vi "QuickDrop Read QDKS INI Info.vi"(8 "error in":errorcluster, 11 "Mappings from INI":string) -> (0 "error out":errorcluster, 1 "All Plugin Paths":path[](array[path]), 2 "INI Names":string[](array[string]), 3 "INI Configured Shortcuts":string[](array[string]))   [LabVIEW 2020]
uses:
  <vilib>/Utility/lvfile.llb/NI_FileType.lvlib
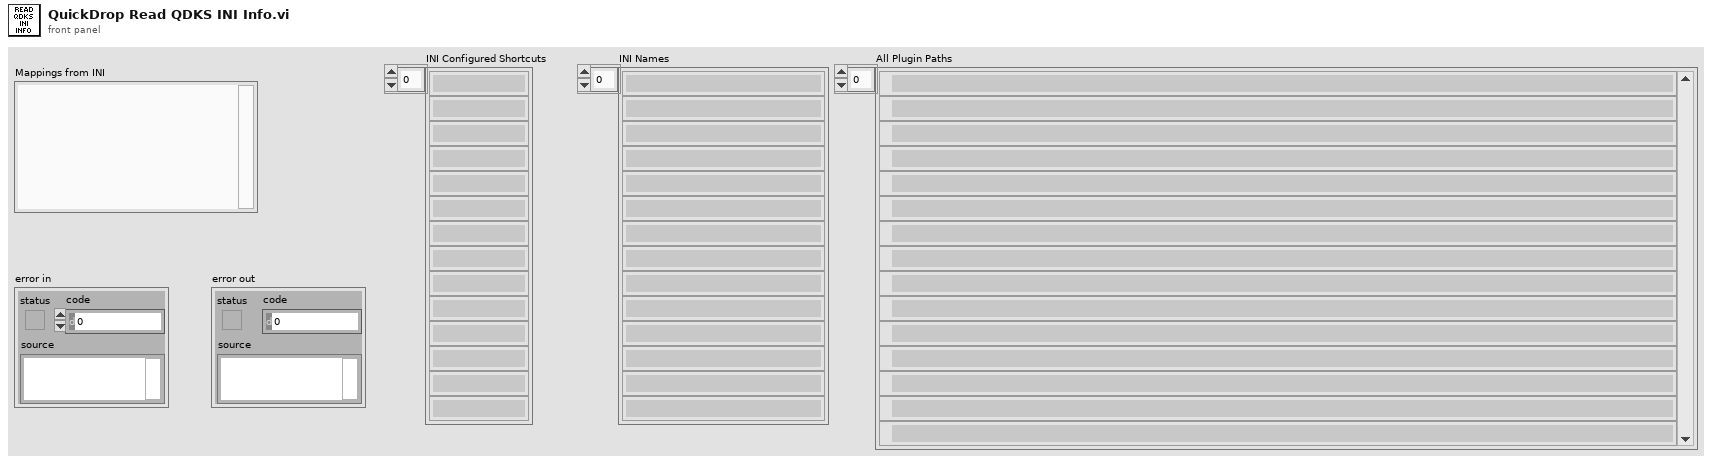
[diagram p1: front panel]
types:
  T1 = typedef "NI_FileType.lvlib/FT_FileTypes.ctl" = enum32{"Invalid file/path", "Unknown type", "Instrument", "Control", "Polymorphic VI", "Project", "Library", "LVClass", "XControl", "XNode", "CIN", "Run-time menu", "Palette menu", "LLB", "Shortcut", "Directory", "Class Private Data Control", "Statechart", "MathScript .m file", "Ladder Diagram", "LVLibp"}
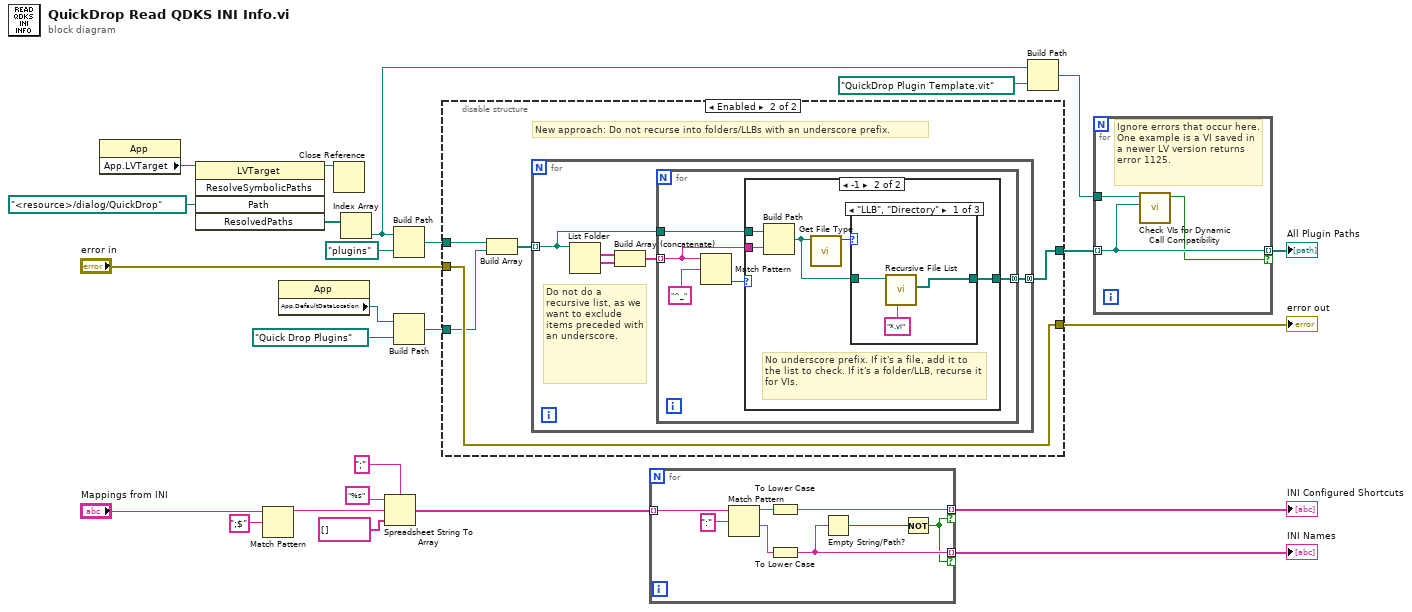
[diagram p0: block diagram]
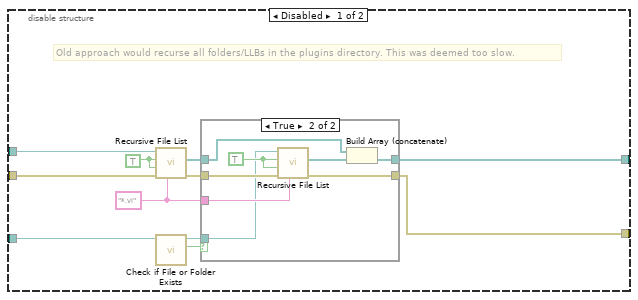
[diagram p2: hidden frame]
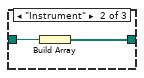
[diagram p5: hidden frame]
diagram:
  n1 = property class="App"() -> ("App.LVTarget"=w5:refnum<vi>)  [unwired: 2 in, 2 out]
  n2 = invoke class="LVTarget" method="ResolveSymbolicPaths"(reference=w5, "Path"=path "<resource>/dialog/QuickDrop") -> (reference out=w3:refnum<vi>, "ResolvedPaths"=w2:path[])  [unwired: 3 in, 3 out]
  n3 = Match Pattern(string="Mappings from INI", regular expression=";$") -> (before substring=w16:string)  [unwired: 1 in, 3 out]
  n4 = property class="App"() -> ("App.DefaultDataLocation"=w13:path)  [unwired: 2 in, 2 out]
  n5 = Close Reference(reference=w3) -> ()  [unwired: 1 in, 1 out]
  n6 = Index Array(array=w2) -> (element=w1:path)  [unwired: 1 in]
  n7 = Spreadsheet String To Array(delimiter (Tab)=";", format string="%s", spreadsheet string=w16, array type (2D Dbl)=string[] []) -> (array=w19:string[])
  n8 = Build Path(base path=w1, name or relative path=path "plugins" ("Application:Directory Path")) -> (appended path=w11:path)
  n9 = Build Path(base path=w13, name or relative path=path "Quick Drop Plugins" ("Application:Directory Path")) -> (appended path=w20:path)
  n10 = disable-structure shown="Enabled" {
    disable-tunnel: [w36 w51] -> w22
    disable-tunnel: "error in" -> [w35 w51]
    disable-tunnel: w20 -> [w31 w49]
    disable-tunnel: w11 -> [w30 w50]
    disable-tunnel: [w26 w47] -> w9
    frame Disabled {
      w27 = TRUE ("Treat LLBs as Folders?")
      w29 = "*.vi" ("pattern")
      # "Old approach would recurse all folders/LLBs in the plugins directory. This was deemed too slow."
      n11 = call <vilib>:"Recursive File List.vi"("pattern"=w29, "error in (no error)"=w35, "Continue Recursing on Error? (F)"=w27, "Treat LLBs as Folders?"=w27, "Folder Path"=w30) -> ("error out"=w28:errorcluster, "All Files in Dir"=w34:path[])  [unwired: 2 in, 3 out]
      n12 = call <vilib>:"Check if File or Folder Exists.vi"("path"=w31) -> ("file or folder exists?"=w33:bool, "dup path"=w32:path)  [unwired: 8 in, 1 out]
      n13 = case shown="True" w33 {
        tunnel: w28 -> [w38 w46]
        tunnel: w29 -> [_ w44]
        tunnel: [w37 w40] -> w26
        tunnel: [w38 w42] -> w36
        tunnel: w32 -> [_ w41]
        tunnel: w34 -> [w37 w39]
        frame False {
        }
        frame True {
          w45 = TRUE ("Treat LLBs as Folders?")
          n14 = call <vilib>:"Recursive File List.vi"("pattern"=w44, "error in (no error)"=w46, "Continue Recursing on Error? (F)"=w45, "Treat LLBs as Folders?"=w45, "Folder Path"=w41) -> ("error out"=w42:errorcluster, "All Files in Dir"=w43:path[])  [unwired: 2 in, 3 out]
          n15 = Build Array (concatenate)(w39, w43) -> (w40:path[])
        }
      }
    }
    frame Enabled {
      # "New approach: Do not recurse into folders/LLBs with an underscore prefix."
      n16 = Build Array(w50, w49) -> (w48:path[])
      n17 = for {
        tunnel: w48 -> [w53] mode=indexing
        tunnel: [w52] -> w47 mode=concatenating
        # "Do not do a recursive list, as we want to exclude items preceded with an underscore."
        n18 = List Folder(path=w53) -> (filenames=w56:string[], folder names=w55:string[])  [unwired: 3 in, 2 out]
        n19 = Build Array (concatenate)(w56, w55) -> (w54:string[])
        n20 = for {
          tunnel: w54 -> [w58] mode=indexing
          tunnel: w53 -> [w59]
          tunnel: [w57] -> w52 mode=concatenating
          n21 = Match Pattern(string=w58, regular expression="^_") -> (offset past match=w60:i32)  [unwired: 1 in, 3 out]
          n22 = case shown="-1" w60 {
            tunnel: w59 -> [_ w66]
            tunnel: w58 -> [_ w65]
            tunnel: [_ w62] -> w57
            frame Default {
              # "This item name is preceded with an underscore. Do not consider it as a plugin, and if it's a folder/LLB, do not recurse into it."
            }
            frame -1 {
              # "No underscore prefix. If it's a file, add it to the list to check. If it's a folder/LLB, recurse it for VIs."
              n23 = Build Path(base path=w66, name or relative path=w65) -> (appended path=w63:path)
              n24 = call <vilib>:"Get File Type.vi"("path"=w63) -> ("file type"=w64:T1)  [unwired: 8 in, 2 out]
              n25 = case shown="\"LLB\", \"Directory\"" w64 {
                tunnel: w63 -> [w69 w71 _]
                tunnel: [w68 w70 _] -> w62
                frame "LLB", "Directory" {
                  n26 = call <vilib>:"Recursive File List.vi"("pattern"="*.vi", "Folder Path"=w69) -> ("All Files in Dir"=w68:path[])  [unwired: 5 in, 4 out]
                }
                frame "Instrument" {
                  n27 = Build Array(w71) -> (w70:path[])
                }
                frame Default {
                }
              }
            }
          }
        }
      }
    }
  }
  "error out" <- w22
  n28 = for {
    tunnel: w19 -> [w79] mode=indexing
    tunnel: [w75] -> w25 mode=indexing if=w73
    tunnel: [w74] -> w24 mode=indexing if=w73
    n29 = Match Pattern(string=w79, regular expression=":") -> (before substring=w77:string, after substring=w76:string)  [unwired: 1 in, 2 out]
    n30 = To Lower Case(string=w77) -> (all lower case string=w75:string)
    n31 = To Lower Case(string=w76) -> (all lower case string=w74:string)
    n32 = Empty String/Path?(string/path=w74) -> (empty?=w72:bool)
    n33 = Not(x=w72) -> (.not. x?=w73:bool)
  }
  "INI Configured Shortcuts" <- w25
  "INI Names" <- w24
  n34 = Build Path(base path=w1, name or relative path=path "QuickDrop Plugin Template.vit" ("Application:Directory Path")) -> (appended path=w7:path)
  n35 = for {
    tunnel: w9 -> [w81] mode=indexing
    tunnel: w7 -> [w82]
    tunnel: [w81] -> w6 mode=indexing if=w80
    # "Ignore errors that occur here. One example is a VI saved in a newer LV version returns error 1125."
    n36 = call <vilib>:"Check VIs for Dynamic Call Compatibility.vi"("VI 2"=w81, "VI 1"=w82) -> ("Compatible for dynamic call?"=w80:bool)  [unwired: 8 in, 1 out]
  }
  "All Plugin Paths" <- w6
